vi "Visa.vi"() -> ()   [LabVIEW 2025]
uses:
  <vilib>/Instr/_visa.llb/VISA Configure Serial Port (Instr).vi
panel:
  out "Temperature":dbl
  in  "Stop Button":bool
  out "Waveform Chart":dbl(graph)
  in  "VISA resource name":refnum<visa-resource-name>
  # "Virtual Instrument LAB : VISA Serial"
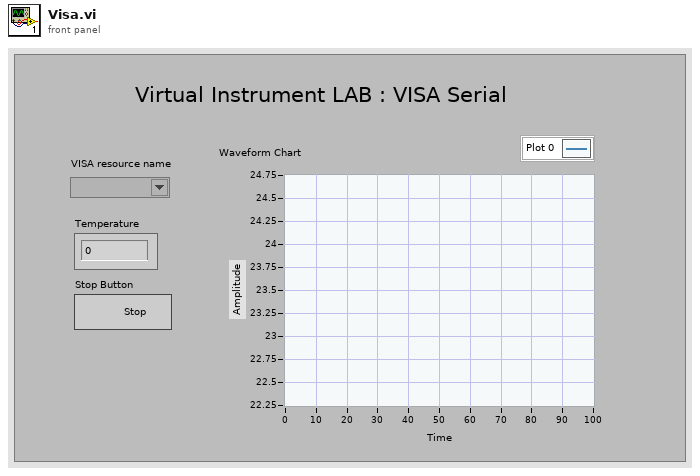
[diagram p1: front panel]
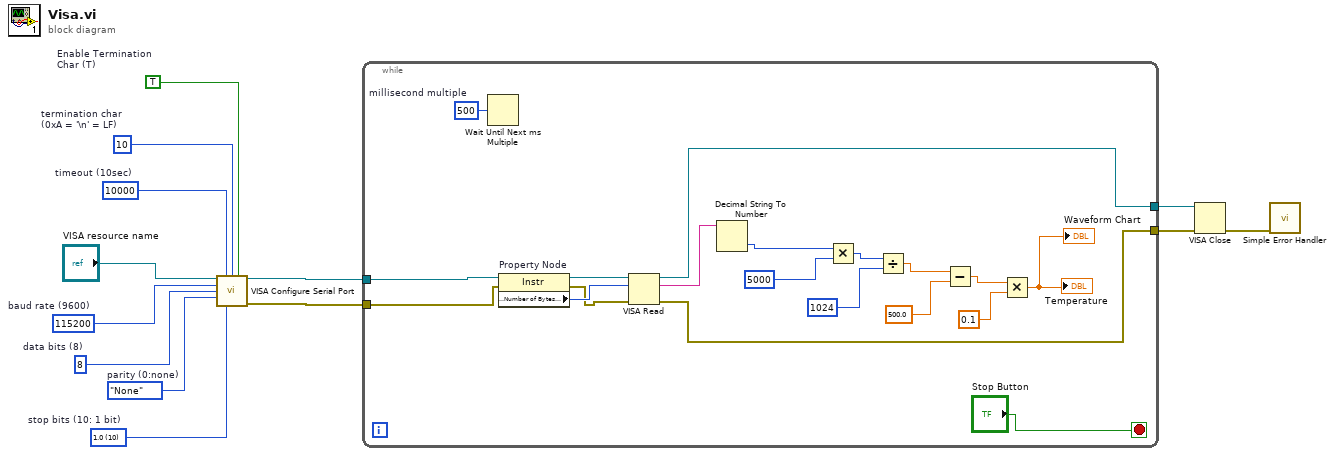
[diagram p0: block diagram]
diagram:
  w6 = u16 10 items=["1.0"=10, "1.5"=15, "2.0"=20]  # stop bits (10: 1 bit)
  w7 = enum16{"None", "Odd", "Even", "Mark", "Space"}."None"  # parity (0:none)
  w8 = u16 8  # data bits (8)
  w9 = u32 115200  # baud rate (9600)
  w10 = TRUE  # Enable Termination Char (T)
  w11 = u8 10  # termination char (0xA = '\n' = LF)
  w12 = u32 10000  # timeout (10sec)
  n1 = call-poly "VISA Configure Serial Port"("VISA resource name"="VISA resource name", "timeout (10sec)"=w12, "termination char\n(0xA = '\\n' = LF)"=w11, "Enable Termination\nChar (T)"=w10, "baud rate (9600)"=w9, "data bits (8)"=w8, "parity (0:none)"=w7, "stop bits (10: 1 bit)"=w6) -> ("VISA resource name out"=w5:refnum<visa-resource-name>, "error out"=w4:errorcluster)  [unwired: 6 in]
  n2 = while {
    tunnel: w5 -> [w31]
    tunnel: w4 -> [w30]
    tunnel: [w17] -> w3
    tunnel: [w16] -> w2
    stop <- "Stop Button" stop-if-true
    w32 = u32 500  # millisecond multiple
    n3 = Wait Until Next ms Multiple(millisecond multiple=w32) -> ()  [unwired: 1 out]
    n4 = property on="Property Node" class="Instr"(reference=w31, error in=w30) -> (reference out=w29:refnum<visa-resource-name>, error out=w27:errorcluster, "Serial Settings:Number of Bytes at Serial Port"=w28:u32)
    n5 = VISA Read(VISA resource name=w29, byte count=w28, error in (no error)=w27) -> (VISA resource name out=w17:refnum<visa-resource-name>, read buffer=w26:string, error out=w16:errorcluster)  [unwired: 1 out]
    n6 = Decimal String To Number(string=w26) -> (number=w25:i32)  [unwired: 2 in, 1 out]
    n7 = Multiply(x=w25, y=5000) -> (x*y=w23:i32)
    n8 = Divide(x=w23, y=1024) -> (x/y=w21:dbl)
    n9 = Subtract(x=w21, y=500.0) -> (x-y=w19:dbl)
    n10 = Multiply(x=w19, y=0.1) -> (x*y=→"Waveform Chart" →"Temperature":dbl)
  }
  n11 = VISA Close(VISA resource name=w3, error in (no error)=w2) -> (error out=w1:errorcluster)
  n12 = call <vilib>:"Simple Error Handler.vi"("error in (no error)"=w1) -> ()  [unwired: 4 in, 5 out]
